vi "sygnalizator.vi"() -> ()   [LabVIEW 2018]
panel:
  in  "pause":bool
  in  "stop":bool
  out "Cluster":T1
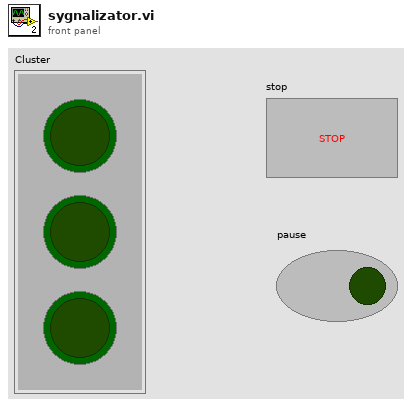
[diagram p1: front panel]
types:
  T1 = cluster{"czerwone":bool, "¿ó³te":bool, "zielone ":bool}
  T2 = typedef "œwiat³a.ctl" = enum16{"¿ó³te+czerwone", "zielone", "¿ó³te", "czerwone"}
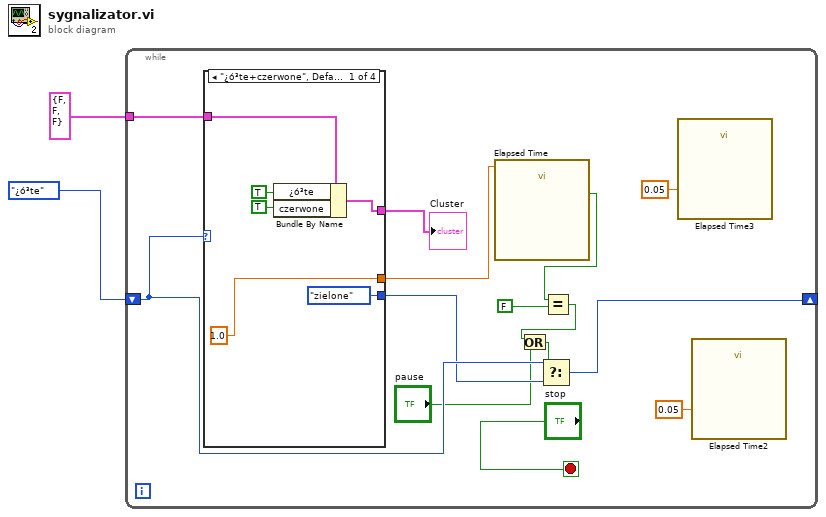
[diagram p0: block diagram]
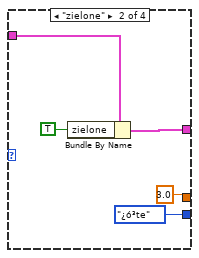
[diagram p2: hidden frame]
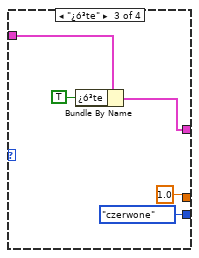
[diagram p3: hidden frame]
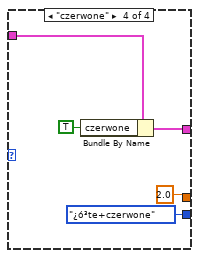
[diagram p4: hidden frame]
diagram:
  n1 = while {
    shift-right: [w10] -> _
    shift-left: œwiat³a."¿ó³te" -> [w13]
    tunnel: T1 {"czerwone"=FALSE, "¿ó³te"=FALSE, "zielone "=FALSE} ("Cluster 2") -> [w14]
    stop <- "stop" stop-if-true
    n2 = case shown="\"¿ó³te+czerwone\", Default" w13 {
      tunnel: [w21 w27 w31 w37] -> w16
      tunnel: [œwiat³a."zielone" œwiat³a."¿ó³te" œwiat³a."czerwone" œwiat³a."¿ó³te+czerwone"] -> w12
      tunnel: w14 -> [w22 w24 w32 w34]
      tunnel: [1.0 ("Time Target (s)") 3.0 ("Time Target (s)") 1.0 ("Time Target (s)") 2.0 ("Time Target (s)")] -> w11
      frame "¿ó³te+czerwone", Default {
        n3 = Bundle By Name(cluster=w22, "¿ó³te"=TRUE, "czerwone"=TRUE) -> (w21:T1)
      }
      frame "zielone" {
        n4 = Bundle By Name(cluster=w24, "zielone"=TRUE ("czerwone")) -> (w27:T1)
      }
      frame "¿ó³te" {
        n5 = Bundle By Name(cluster=w32, "¿ó³te"=TRUE) -> (w31:T1)
      }
      frame "czerwone" {
        n6 = Bundle By Name(cluster=w34, "czerwone"=TRUE) -> (w37:T1)
      }
    }
    "Cluster" <- w16
    n7 = call "Elapsed Time"("Time Target (s)"=w11) -> ("Time has Elapsed"=w9:bool)  [unwired: 11 in, 7 out]
    n8 = Equal?(x=w9, y=FALSE) -> (x = y?=w7:bool)
    n9 = Or(x=w7, y="pause") -> (x .or. y?=w5:bool)
    n10 = Select(t=w13, s=w5, f=w12) -> (s? t:f=w10:T2)
    n11 = call "Elapsed Time3"("Set Start Time (s)"=0.05) -> ()  [unwired: 11 in, 8 out]
    n12 = call "Elapsed Time2"("Set Start Time (s)"=0.05) -> ()  [unwired: 11 in, 8 out]
  }
